vi "TRAJECTORY_CREATE_CUBIC_BEGIN_OLD.vi"() -> (0 "Trajectory \ncalculation \nerror":errorcluster, 2 "Trajectory Items":i32, 3 "TotalTImeSecs":dbl)   [LabVIEW 2019]
uses:
  <vilib>/Rock Robotics/WPI/ThirdParty/JAS_Junk/TrajLib/Rotation_CreateAngle.vi
  <vilib>/Rock Robotics/SystemInterfaces/NetworkCommunication/NetComm_UsageReport_report.vi
  <vilib>/Rock Robotics/WPI/ThirdParty/JAS_Junk/TrajLib/DiffDriveKinematicsConstraint_New.vi
  <vilib>/Rock Robotics/WPI/ThirdParty/JAS_Junk/TrajLib/CentripetalAccelConstraint_New.vi
  <vilib>/Rock Robotics/WPI/ThirdParty/JAS_Junk/TrajLib/Util_LibraryGlobals.vi
  <vilib>/Rock Robotics/WPI/ThirdParty/JAS_Junk/TrajLib/Trajectory_Library.lvlib
panel:
  in  "Interior WayPoints":cluster{"X Inches":dbl, "Y Inches":dbl}[](array[cluster])=[{"X Inches"=105.0, "Y Inches"=65.0}]
  in  "Output Position":T1={"X Inches"=210.0, "Y Inches"=106.0, "Heading\nDegrees"=45.0}
  in  "Input Position":T1={"X Inches"=15.0, "Y Inches"=105.0, "Heading\nDegrees"=-45.0}
  in  "Use Diff Drive\nKinematic\nConstraint":bool=TRUE
  in  "Use Centripetal\nAcceleration\nConstaint":bool=TRUE
  out "Wheelbase Width":dbl=0.66 format="%20.4f"
  out "MaxAcceleration":dbl=1.3 format="%17.4f"
  out "MaxVelocity":dbl=2.0 format="%17.4f"
  out "Max Cent Accel":dbl=1.0 format="%20.4f"
  in  "Max Cent Accel INCHES/SEC^2":dbl=7.0 format="%20.1f"
  in  "MaxAcceleration INCHES/SEC^2":dbl=35.0 format="%17.1f"
  in  "MaxVelocity Fraction":dbl=0.66 format="%17.3f"
  # "TRAJECTORY CONFIGURATION"
  # "real 20.9 inch"
  # "TRAJECTORY DEFINITION"
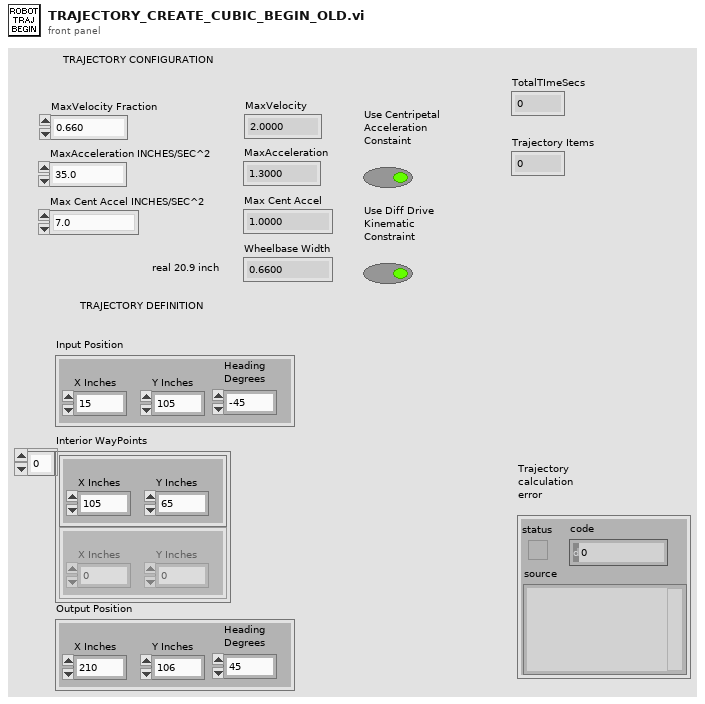
[diagram p1: front panel]
types:
  T1 = cluster{"X Inches":dbl, "Y Inches":dbl, "Heading\nDegrees":dbl}
  T2 = typedef "Trajectory_Library.lvlib/TRANSLATION2D.ctl" = cluster{"X":dbl, "Y":dbl}
  T3 = typedef "Trajectory_Library.lvlib/POSE2D.ctl" = cluster{"TRANSLATION":T2, "ROTATION":T4}
  T4 = typedef "Trajectory_Library.lvlib/ROTATION2D.ctl" = cluster{"VALUE":dbl, "COS":dbl, "SIN":dbl}
  T5 = typedef "Trajectory_Library.lvlib/TRAJ_CONFIG.ctl" = cluster{"MaxVelocity":dbl, "Max Acceleration":dbl, "StartVelocity":dbl, "End Velocity":dbl, "Reversed":bool, "DiffDrKineConstntDefined":bool, "CentAcellConstntDefined":bool, "DiffDrVoltConstntDefined":bool, "DIFF_DRIVE_KINE_CONSTRAINT":T6, "CENTRIPETAL_ACCEL_CONSTRAINT":T8, "SwerveDrKineConstntDefined":bool, "SWERVE_DRIVE_KINE_CONSTRAINT":T9, "DIFF_DRIVE_VOLTAGE_CONSTRAINT":T12, "MECANUM_DRIVE_KINE_CONSTRAINT":T14, "MecanumDrKineConstntDefined":bool}
  T6 = typedef "Trajectory_Library.lvlib/TRAJ_CONSTRAINT_DIIF_DRIVE_KINEMATICS.ctl" = cluster{"Max Speed (M/S)":dbl, "DIFF_DRIVE_KINEMATICS":T7}
  T7 = typedef "Trajectory_Library.lvlib/DIFF_DRIVE_KINEMATICS.ctl" = cluster{"TrackWidth_Meters":dbl}
  T8 = typedef "Trajectory_Library.lvlib/TRAJ_CONSTRAINT_CENTRIPETAL_ACCEL.ctl" = cluster{"Max Cent Accel":dbl}
  T9 = typedef "Trajectory_Library.lvlib/TRAJ_CONSTRAINT_SWERVE_DRIVE_KINEMATICS.ctl" = cluster{"Max Speed (M/S)":dbl, "SwerveKinematics":T10}
  T10 = typedef "Trajectory_Library.lvlib/SWERVE_DRIVE_KINEMATICS.ctl" = cluster{"NumModules":i32, "InverseKinematics":T11, "ForwardKinematics":T11, "Modules":T2[], "PrevCoR":T2}
  T11 = typedef "NI_Matrix.lvlib/RealMatrix.ctl" = dbl[][]
  T12 = typedef "Trajectory_Library.lvlib/TRAJ_CONSTRAINT_DIIF_DRIVE_VOLTAGE.ctl" = cluster{"Max Voltage":dbl, "DIFF_DRIVE_KINEMATICS":T7, "SIMPLE_MOTOR_FF":T13}
  T13 = typedef "Trajectory_Library.lvlib/SIMPLE_MOTOR_FF.ctl" = cluster{"Ks":dbl, "Kv":dbl, "Ka":dbl}
  T14 = typedef "Trajectory_Library.lvlib/TRAJ_CONSTRAINT_MECA_DRIVE_KINEMATICS.ctl" = cluster{"Max Speed (M/S)":dbl, "MECA_DRIVE_KINEMATICS":T15}
  T15 = typedef "Trajectory_Library.lvlib/MECA_DRIVE_KINEMATICS.ctl" = cluster{"FrontLeft":T2, "FrontRight":T2, "RearLeft":T2, "RearRight":T2, "InverseKinematics":T11, "ForwardKinematics":T11, "PrevCoR":T2}
  T16 = typedef "Trajectory_Library.lvlib/TRAJECTORY.ctl" = cluster{"TotalTImeSecs":dbl, "States":T17[]}
  T17 = typedef "Trajectory_Library.lvlib/TRAJ_STATE.ctl" = cluster{"TimeSeconds":dbl, "Velocity":dbl, "Acceleration":dbl, "POSE":T3, "Curvature":dbl}
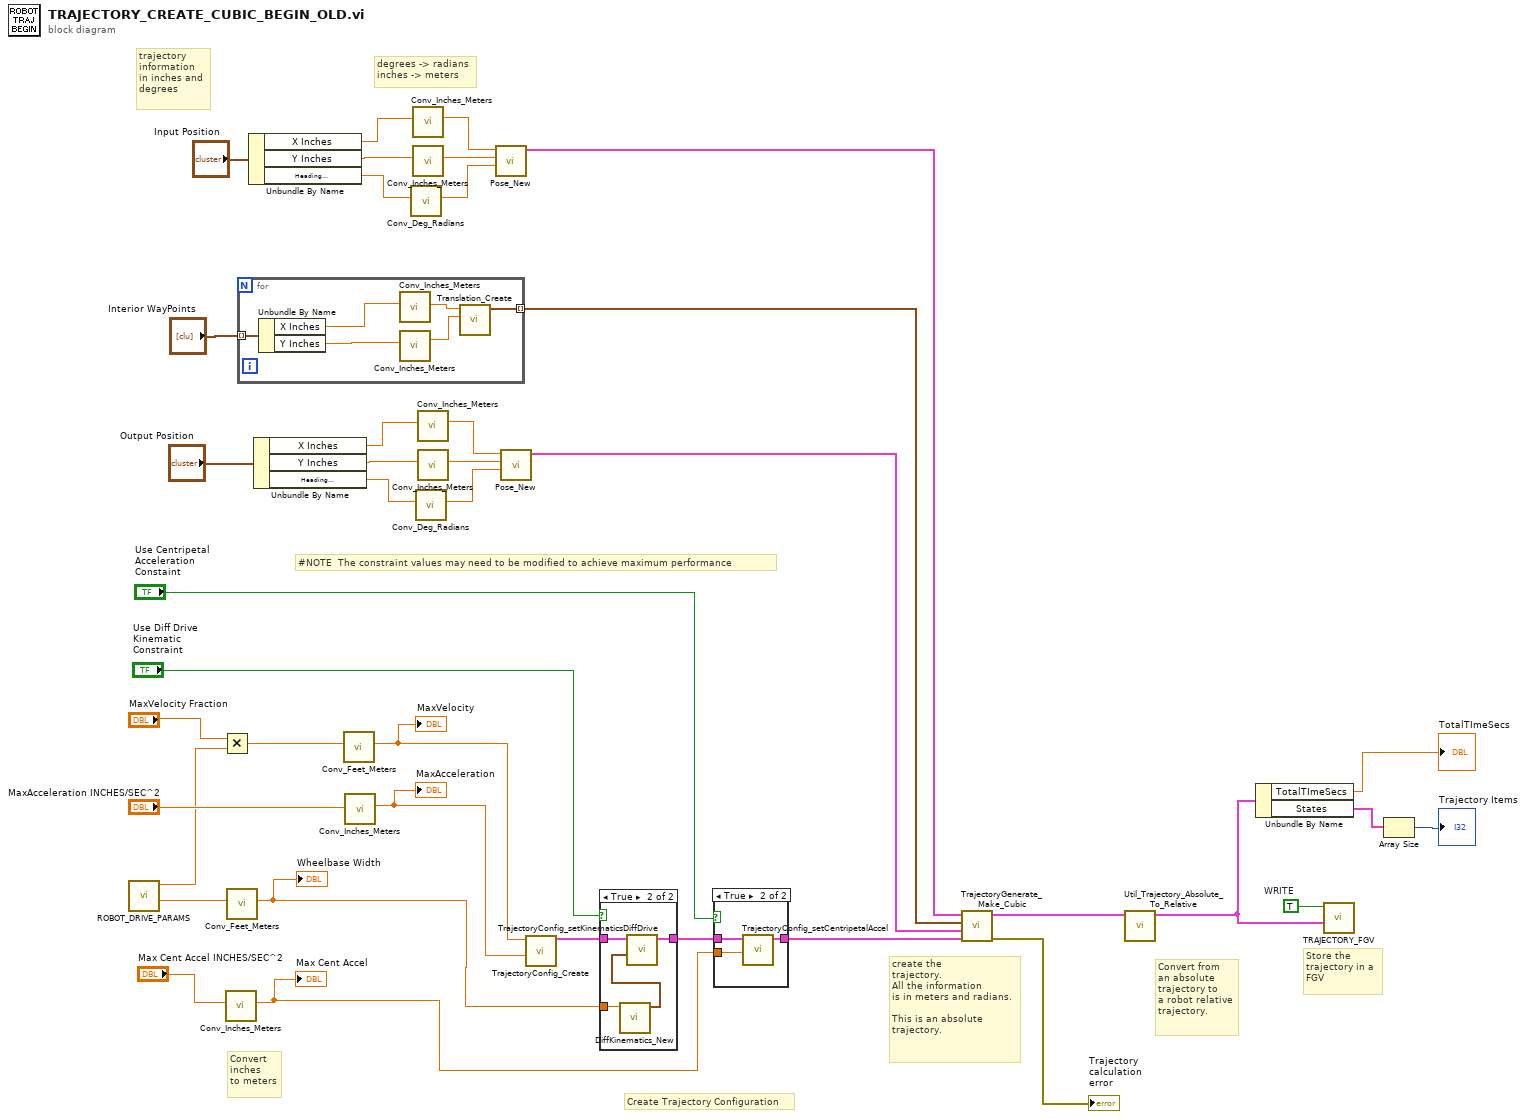
[diagram p0: block diagram]
diagram:
  w10 = TRUE  # WRITE
  # "#NOTE  The constraint values may need to be modified to achieve maximum performance"
  # "Store the\ntrajectory in a \nFGV"
  # "Convert from\nan absolute\ntrajectory to\na robot relative\ntrajectory."
  # "Convert\ninches\nto meters"
  # "degrees -> radians\ninches -> meters"
  # "create the\ntrajectory.\nAll the information\nis in meters and radians.\n\nThis is an absolute \ntrajectory."
  # "trajectory\ninformation\nin inches and\ndegrees"
  # "Create Trajectory Configuration"
  n1 = call "ROBOT_DRIVE_PARAMS.vi"() -> ("Effective Wheelbase Ft"=w4:dbl, "Max Speed Ft/Sec"=w1:dbl)  [unwired: 10 in]
  n2 = Multiply(x="MaxVelocity Fraction", y=w1) -> (x*y=w3:dbl)
  n3 = call <vilib>:"Conv_Inches_Meters.vi"("INCH"="Max Cent Accel INCHES/SEC^2") -> ("Meters"=w33:dbl)  [unwired: 10 in]
  "Max Cent Accel" <- w33
  n4 = call <vilib>:"Conv_Feet_Meters.vi"("Feet"=w4) -> ("Meters"=w34:dbl)  [unwired: 10 in]
  "Wheelbase Width" <- w34
  n5 = for {
    tunnel: "Interior WayPoints" -> [w44] mode=indexing
    tunnel: [w41] -> w12 mode=indexing
    n6 = Unbundle By Name(w44) -> ("X Inches"=w46:dbl, "Y Inches"=w45:dbl)
    n7 = call <vilib>:"Conv_Inches_Meters.vi"("INCH"=w46) -> ("Meters"=w43:dbl)  [unwired: 10 in]
    n8 = call <vilib>:"Conv_Inches_Meters.vi"("INCH"=w45) -> ("Meters"=w42:dbl)  [unwired: 10 in]
    n9 = call <vilib>:"Translation_Create.vi"("Y"=w42, "X"=w43) -> ("TRANSLATION"=w41:T2)  [unwired: 9 in]
  }
  n10 = Unbundle By Name("Input Position") -> ("X Inches"=w27:dbl, "Y Inches"=w26:dbl, "Heading\nDegrees"=w24:dbl)
  n11 = Unbundle By Name("Output Position") -> ("X Inches"=w20:dbl, "Y Inches"=w19:dbl, "Heading\nDegrees"=w17:dbl)
  n12 = call <vilib>:"Conv_Feet_Meters.vi"("Feet"=w3) -> ("Meters"=w31:dbl)  [unwired: 10 in]
  "MaxVelocity" <- w31
  n13 = call <vilib>:"Conv_Inches_Meters.vi"("INCH"="MaxAcceleration INCHES/SEC^2") -> ("Meters"=w32:dbl)  [unwired: 10 in]
  "MaxAcceleration" <- w32
  n14 = call <vilib>:"Conv_Deg_Radians.vi"("Degress"=w24) -> ("Radians"=w25:dbl)  [unwired: 10 in]
  n15 = call <vilib>:"Conv_Inches_Meters.vi"("INCH"=w27) -> ("Meters"=w22:dbl)  [unwired: 10 in]
  n16 = call <vilib>:"Conv_Inches_Meters.vi"("INCH"=w26) -> ("Meters"=w23:dbl)  [unwired: 10 in]
  n17 = call <vilib>:"Conv_Deg_Radians.vi"("Degress"=w17) -> ("Radians"=w18:dbl)  [unwired: 10 in]
  n18 = call <vilib>:"Conv_Inches_Meters.vi"("INCH"=w20) -> ("Meters"=w15:dbl)  [unwired: 10 in]
  n19 = call <vilib>:"Conv_Inches_Meters.vi"("INCH"=w19) -> ("Meters"=w16:dbl)  [unwired: 10 in]
  n20 = call <vilib>:"Pose_New.vi"("Heading"=w25, "Y"=w23, "X"=w22) -> ("out POSe"=w11:T3)  [unwired: 8 in]
  n21 = call <vilib>:"Pose_New.vi"("Heading"=w18, "Y"=w16, "X"=w15) -> ("out POSe"=w13:T3)  [unwired: 8 in]
  n22 = call <vilib>:"TrajectoryConfig_Create.vi"("MaxAcceleration"=w32, "MaxVelocity"=w31) -> ("TRAJECTORY_CONFIG"=w38:T5)  [unwired: 9 in]
  n23 = case shown="True" "Use Diff Drive\nKinematic\nConstraint" {
    tunnel: w38 -> [w47 w51]
    tunnel: [w47 w50] -> w37
    tunnel: w34 -> [_ w48]
    frame False {
    }
    frame True {
      n24 = call <vilib>:"DiffKinematics_New.vi"("TrackWidth_Meters"=w48) -> ("DIFF_DRIVE_KINEMATICS"=w49:T7)  [unwired: 10 in]
      n25 = call <vilib>:"TrajectoryConfig_setKinematicsDiffDrive.vi"("DIFF_DRIVE_KINEMATICS"=w49, "inTRAJECTORY_CONFIG"=w51) -> ("outTRAJECTORY_CONFIG"=w50:T5)  [unwired: 9 in]
    }
  }
  n26 = case shown="True" "Use Centripetal\nAcceleration\nConstaint" {
    tunnel: w37 -> [w52 w55]
    tunnel: [w52 w54] -> w29
    tunnel: w33 -> [_ w53]
    frame False {
    }
    frame True {
      n27 = call <vilib>:"TrajectoryConfig_setCentripetalAccel.vi"("Max Cent Accel"=w53, "inTRAJECTORY_CONFIG"=w55) -> ("outTRAJECTORY_CONFIG"=w54:T5)  [unwired: 9 in]
    }
  }
  n28 = call <vilib>:"TrajectoryGenerate_Make_Cubic.vi"("traj_config"=w29, "Enging POSE"=w13, "Interior WAYPOINTS"=w12, "Starting POSE"=w11) -> ("error out"=→"Trajectory \ncalculation \nerror":errorcluster, "TRAJECTORY"=w5:T16)  [unwired: 6 in]
  n29 = call <vilib>:"Util_Trajectory_Absolute_To_Relative.vi"("absTRAJECTORY"=w5) -> ("outputRelativeTRAJECTORY"=w6:T16)  [unwired: 10 in]
  n30 = Unbundle By Name(w6) -> ("TotalTImeSecs"=→"TotalTImeSecs":dbl, "States"=w8:T17[])
  n31 = call "TRAJECTORY_FGV.vi"("inTRAJECTORY"=w6, "WRITE"=w10) -> ()  [unwired: 9 in, 1 out]
  n32 = Array Size(array=w8) -> (size(s)=→"Trajectory Items":i32)
